vi "Write DCM Ref.vi"(8 "error in (no error)":errorcluster, 10 "DCM Ref":refnum<class "DCM - RT.lvclass">, 11 "DCM-DSI-HW in":refnum<class "DCM-DSI.lvclass">) -> (0 "error out":errorcluster, 3 "DCM-DSI-HW out":refnum<class "DCM-DSI.lvclass">)   [LabVIEW 2016, in "DCM-DSI.lvclass"]
uses:
  DCM-DSI.lvclass
  <vilib>/Powertrain Controls/Device Drivers/DCM/Rev0/RT/DCM - RT.lvclass
  DCM-DSI.lvclass/DCM-DSI.ctl
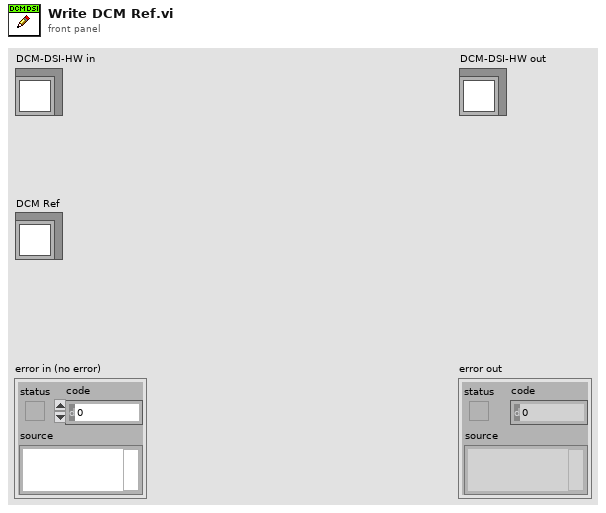
[diagram p1: front panel]
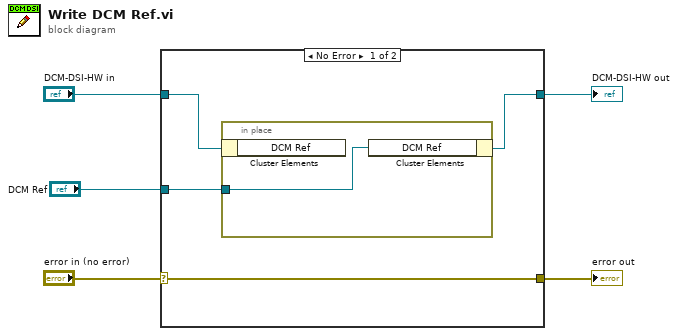
[diagram p0: block diagram]
diagram:
  n1 = case shown="No Error" "error in (no error)" {
    selector: "error in (no error)" -> [w6 w11]
    tunnel: "DCM-DSI-HW in" -> [w9 w12]
    tunnel: [w8 w12] -> w4
    tunnel: "DCM Ref" -> [w7 _]
    tunnel: [w6 w11] -> w1
    frame No Error {
      n2 = in-place {
        in-place-border: w7 -> [w10]
        n3 = in-place-cluster #1(w9) -> ()  [unwired: 1 out]
        n4 = in-place-cluster #1("DCM Ref"=w10) -> (w8:refnum<class "DCM-DSI.lvclass">)
      }
    }
    frame Error {
    }
  }
  "error out" <- w1
  "DCM-DSI-HW out" <- w4
